vi "Main RT.vi"   [LabVIEW 2019]
uses:
  <vilib>/FPGAPlugInAG/sbRIO-9636/niLvFpga_Open_sbRIO-9636.vi
  <vilib>/rvi/interface/common/dynamic/niFpgaDynamicAddResources.vi
  <vilib>/FPGAPlugInAG/Dynamic/niLvFpga_Reset_Dynamic.vi
  <vilib>/FPGAPlugInAG/Dynamic/niLvFpga_Run_Dynamic.vi
  <vilib>/Utility/error.llb/Error Cluster From Error Code.vi
  <vilib>/rvi/errors/niLvFpgaAdjustHostInterfaceError.vi
  <vilib>/FPGAPlugInAG/Dynamic/niLvFpga_Close_Dynamic.vi
  <vilib>/rvi/interface/nirviOpenFPGA/nirviOpenFPGA.xnode
  FPGA Bitfiles/lcddriver_FPGATarget.lvbitx
  Main FPGA.vi
  <vilib>/rvi/interface/nirviMethod/nirviMethod.xnode
  <vilib>/rvi/interface/nirviReadWriteControl/nirviReadWriteControl.xnode
  <vilib>/rvi/interface/nirviCloseFPGA/nirviCloseFPGA.xnode
  HD44780/HD44780.lvlib
  NiFpgaLv.dll
  <vilib>/rvi/interface/Simulation/niFpgaSimulationCallBeginRW.vi
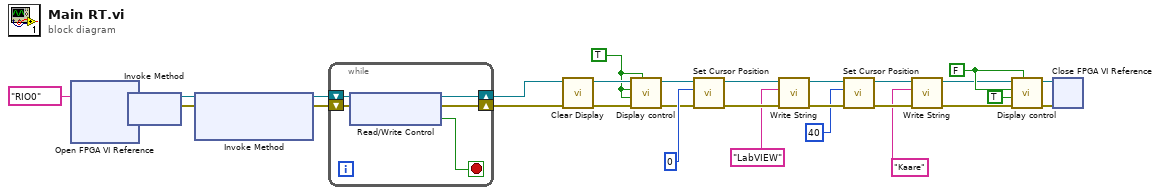
[diagram p0: block diagram]
diagram:
  w1 = TRUE ("Cursor Blink")
  w7 = FALSE ("Cursor Blink")
  n1 = xnode "Open FPGA VI Reference"("resource name"=tag "RIO0") -> ("FPGA VI Reference Out"=w30:refnum<k20>, "error out"=w29:errorcluster)  [unwired: 1 in]
  n2 = xnode "Invoke Method"("FPGA VI Reference In"=w30, "error in"=w29) -> ("FPGA VI Reference Out"=w28:refnum<k20>, "error out"=w27:errorcluster)
  n3 = xnode "Invoke Method"("FPGA VI Reference In"=w28, "error in"=w27) -> ("FPGA VI Reference Out"=w26:refnum<k20>, "error out"=w24:errorcluster)  [unwired: 1 in]
  n4 = while {
    shift-right: [w32] -> w16
    shift-left: w26 -> [w35]
    shift-right: [w33] -> w17
    shift-left: w24 -> [w34]
    stop <- w31 stop-if-true
    n5 = xnode "Read/Write Control"("FPGA VI Reference In"=w35, "error in"=w34) -> ("FPGA VI Reference Out"=w32:refnum<k20>, "error out"=w33:errorcluster, "Display Ready"=w31:bool)
  }
  n6 = call "Clear Display.vi"("error in (no error)"=w17, "Refnum in"=w16) -> ("error out"=w14:errorcluster, "Refnum out"=w15:refnum<k20>)  [unwired: 8 in]
  n7 = call "Display control.vi"("Cursor Blink"=w1, "error in (no error)"=w14, "Enable Display"=w1, "Enable Cursor"=w1, "Refnum in"=w15) -> ("error out"=w21:errorcluster, "Refnum out"=w23:refnum<k20>)  [unwired: 5 in]
  n8 = call "Set Cursor Position.vi"("error in (no error)"=w21, "Position"=u8 0, "Refnum in"=w23) -> ("error out"=w19:errorcluster, "Refnum out"=w20:refnum<k20>)  [unwired: 7 in]
  n9 = call "Write String.vi"("error in (no error)"=w19, "String"="LabVIEW", "Refnum in"=w20) -> ("error out"=w10:errorcluster, "Refnum out"=w12:refnum<k20>)  [unwired: 7 in]
  n10 = call "Set Cursor Position.vi"("error in (no error)"=w10, "Position"=u8 40, "Refnum in"=w12) -> ("error out"=w11:errorcluster, "Refnum out"=w13:refnum<k20>)  [unwired: 7 in]
  n11 = call "Write String.vi"("error in (no error)"=w11, "String"="Kaare", "Refnum in"=w13) -> ("error out"=w2:errorcluster, "Refnum out"=w5:refnum<k20>)  [unwired: 7 in]
  n12 = call "Display control.vi"("Cursor Blink"=w7, "error in (no error)"=w2, "Enable Display"=TRUE, "Enable Cursor"=w7, "Refnum in"=w5) -> ("error out"=w4:errorcluster, "Refnum out"=w3:refnum<k20>)  [unwired: 5 in]
  n13 = xnode "Close FPGA VI Reference"("FPGA VI Reference In"=w3, "error in"=w4) -> ()  [unwired: 1 out]
